vi "destroy by queue.vi"(8 "error in":errorcluster, 10 "timeout in ms (-1)":i32=-1, 11 "queue":refnum<class "identifying queue.lvclass">) -> (0 "error out":errorcluster, 1 "timed out?":bool)   [LabVIEW 2015, in "communicator.lvclass"]
uses:
  communicator.lvclass
  communicator queue/identifying queue.lvclass
  communicator queue/enqueue variety.ctl
  communicator queue/identifying queue.lvclass/identifying queue.ctl
  message/set sender.vi
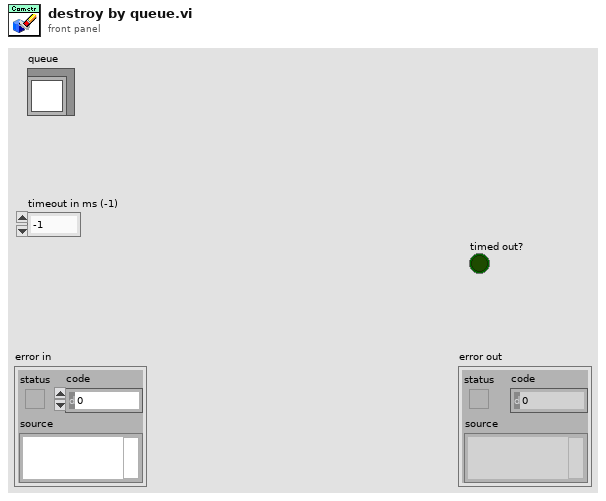
[diagram p1: front panel]
types:
  T1 = typedef "identifying queue.lvclass/enqueue variety.ctl" = enum16{"normal", "lossy", "priority"}
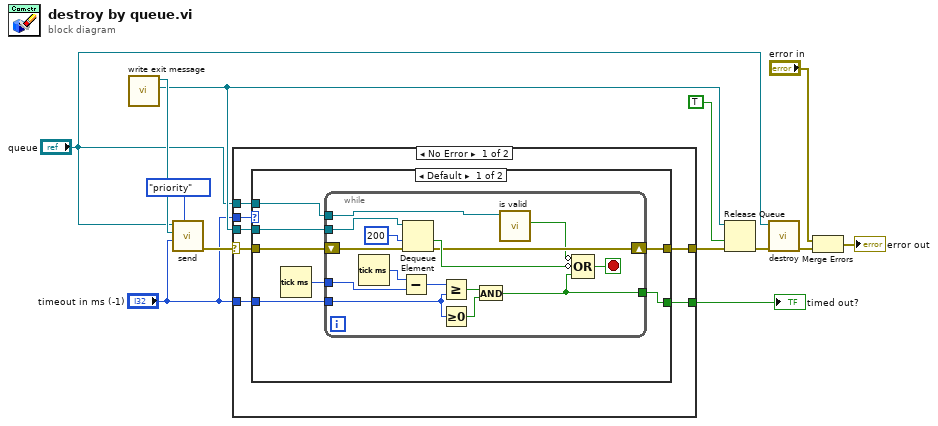
[diagram p0: block diagram]
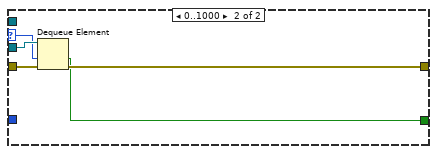
[diagram p2: hidden frame]
diagram:
  n1 = call "write exit message.vi"() -> ("queue out"=w6:refnum<queue>, "message"=w13:refnum<class "communicator message.lvclass">)  [unwired: 10 in]
  n2 = call "send.vi"("enqueue command"=enqueue_variety."priority", "timeout in ms (-1)"="timeout in ms (-1)", "message"=w13, "message connection in"="queue") -> ("error out"=w5:errorcluster)  [unwired: 6 in, 1 out]
  n3 = case shown="No Error" w5 {
    selector: w5 -> [w16 w48]
    tunnel: [w20 w48] -> w11
    tunnel: "timeout in ms (-1)" -> [w19 _]
    tunnel: "queue" -> [w18 _]
    tunnel: w6 -> [w17 _]
    tunnel: "timeout in ms (-1)" -> [w15 _]
    tunnel: [w14 _] -> w1
    frame No Error {
      n4 = case shown="Default" w19 {
        selector: w19 -> [_ w44]
        tunnel: w16 -> [w22 w47]
        tunnel: [w23 w46] -> w20
        tunnel: w17 -> [w26 w45]
        tunnel: w18 -> [w25 _]
        tunnel: w15 -> [w24 _]
        tunnel: [w21 w43] -> w14
        frame Default {
          n5 = Tick Count (ms)() -> (millisecond timer value=w27:u32)
          n6 = while {
            tunnel: w27 -> [w41]
            tunnel: w26 -> [w40]
            tunnel: w25 -> [w31]
            tunnel: w24 -> [w37]
            shift-right: [w30] -> w23
            shift-left: w22 -> [w33]
            tunnel: [w28] -> w21
            stop <- w34 stop-if-true
            n7 = Tick Count (ms)() -> (millisecond timer value=w42:u32)
            n8 = Subtract(x=w42, y=w41) -> (x-y=w39:u32)
            n9 = Dequeue Element(queue=w40, timeout in ms (-1)=u32 200 ("millisecond multiple"), error in (no error)=w33) -> (timed out?=w35:bool, error out=w30:errorcluster)  [unwired: 2 out]
            n10 = Greater Or Equal?(x=w39, y=w37) -> (x >= y?=w38:bool)
            n11 = Greater Or Equal To 0?(x=w37) -> (x >= 0?=w36:bool)
            n12 = And(x=w38, y=w36) -> (x .and. y?=w28:bool)
            n13 = call "is valid.vi"("identifying queue in"=w31) -> ("valid?"=w29:bool)  [unwired: 9 in, 1 out]
            n14 = Compound Arithmetic op=OR(invert w29, invert w35, w28) -> (w34:bool)
          }
        }
        frame 0..1000 {
          n15 = Dequeue Element(queue=w45, timeout in ms (-1)=w44, error in (no error)=w47) -> (timed out?=w43:bool, error out=w46:errorcluster)  [unwired: 2 out]
        }
      }
    }
    frame Error {
    }
  }
  "timed out?" <- w1
  n16 = Release Queue(queue=w6, force destroy? (F)=TRUE, error in (no error)=w11) -> (error out=w10:errorcluster)  [unwired: 2 out]
  n17 = call "destroy.vi"("error in"=w10, "message connection in"="queue") -> ("error out"=w12:errorcluster)  [unwired: 9 in]
  n18 = Merge Errors("error in", w12) -> (→"error out":errorcluster)
